vi "Example Remote Callback - RemoteStatusA Callback.vi"(4 "RemoteStatusA":refnum<user-event>, 5 "Event Data":T1, 6 "Control Ref":refnum<k24>, 7 "Event Common Data":T2) -> ()   [LabVIEW 2013]
uses:
  C:/tf/play/labview/Tinkerforge.dll
  Tinkerforge.dll
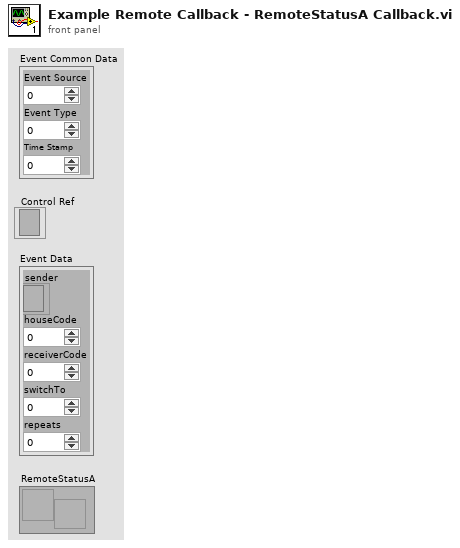
[diagram p1: front panel]
types:
  T1 = cluster{"sender":refnum<k24>, "houseCode":u8, "receiverCode":u8, "switchTo":u8, "repeats":i32}
  T2 = cluster{"Event Source":i32, "Event Type":u32, "Time Stamp":u32}
  T3 = cluster{"houseCode":u8, "receiverCode":u8, "repeats":i32, "switchTo":u8}
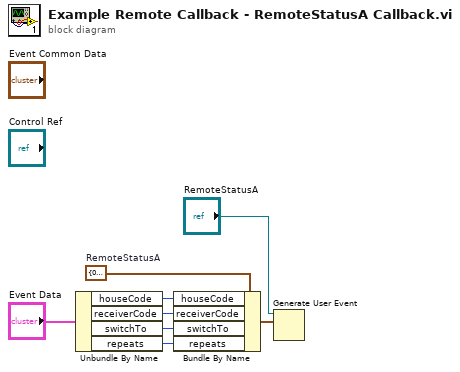
[diagram p0: block diagram]
diagram:
  w7 = T3 {"houseCode"=0, "receiverCode"=0, "repeats"=0, "switchTo"=0}  # RemoteStatusA
  n1 = Unbundle By Name("Event Data") -> ("houseCode"=w6:u8, "receiverCode"=w5:u8, "switchTo"=w4:u8, "repeats"=w3:i32)
  n2 = Bundle By Name(cluster=w7, "houseCode"=w6, "receiverCode"=w5, "switchTo"=w4, "repeats"=w3) -> (w2:T3)
  n3 = Generate User Event(user event="RemoteStatusA", event data cluster=w2) -> ()  [unwired: 2 in, 2 out]
